vi "Get Is Door Open.vi"(8 "error in (no error)":errorcluster, 11 "Door in":refnum<class "Door.lvclass">) -> (0 "error out":errorcluster, 2 "Is Door Open?":bool, 3 "Door out":refnum<class "Door.lvclass">)   [LabVIEW 2018, in "Door.lvclass"]
uses:
  Door.lvclass
  Door.lvclass/Door.ctl
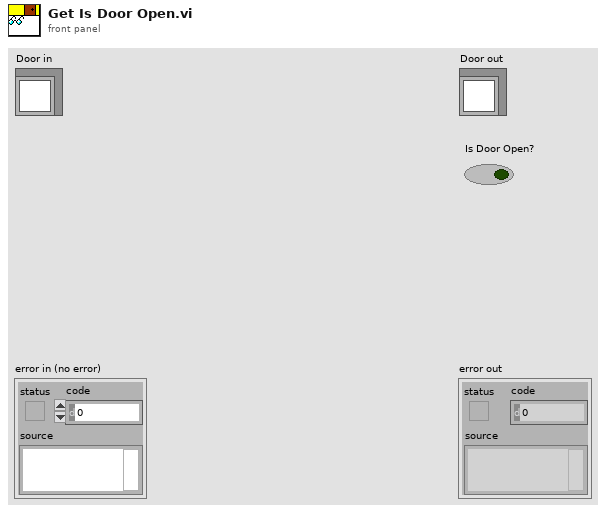
[diagram p1: front panel]
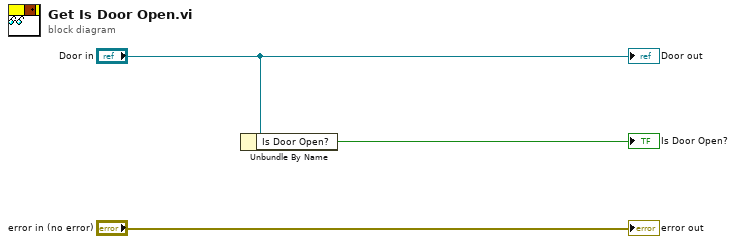
[diagram p0: block diagram]
diagram:
  n1 = Unbundle By Name("Door in") -> ("Is Door Open?"=→"Is Door Open?":bool)
  "error out" <- "error in (no error)"
  "Door out" <- "Door in"
